vi "ziGetValueComplex.vi"(3 "error in":errorcluster, 4 "Path":string, 5 "Handle in":T1 {"Handle" format="0x%08x"; "Conn" format="0x%08x"}) -> (0 "error out":errorcluster, 1 "Value":cdb, 2 "Handle out":T1 {"Handle" format="0x%08x"; "Conn" format="0x%08x"})   [LabVIEW 2019, in "Zurich Instruments LabOne.lvlib"]
doc: "This vi retrieves the numerical value of the specified node as an double-type value. The vi returns the value first found that matches Path if more than one value is available (a wildcard is used in the Path)."
uses:
  Zurich Instruments LabOne.lvlib
  ziTypeHandle.ctl
  Private/ziLV64.dll
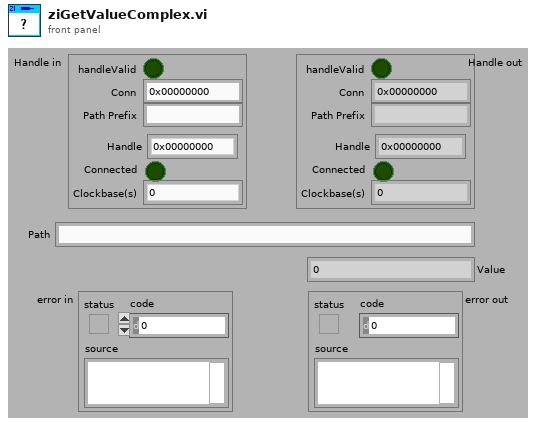
[diagram p1: front panel]
types:
  T1 = typedef "Zurich Instruments LabOne.lvlib/ziTypeHandle.ctl" = cluster{"handleValid":bool, "Conn":u64, "Path Prefix":string, "Handle":u64, "Connected":bool, "Clockbase(s)":dbl}
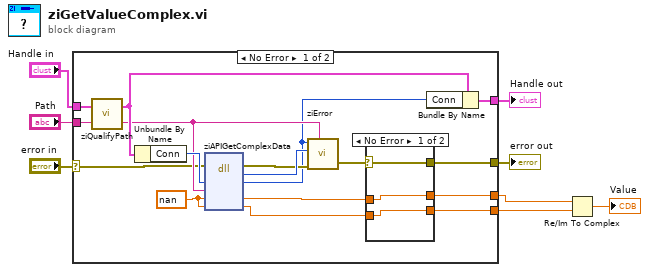
[diagram p0: block diagram]
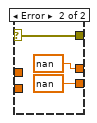
[diagram p2: hidden frame]
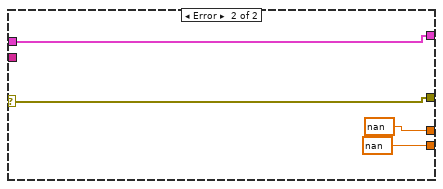
[diagram p3: hidden frame]
diagram:
  n1 = case shown="No Error" "error in" {
    selector: "error in" -> [w16 w35]
    tunnel: [w12 nan ("Value")] -> w2
    tunnel: [w14 w35] -> w8
    tunnel: [w22 w34] -> w7
    tunnel: "Handle in" -> [w21 w34]
    tunnel: "Path" -> [w20 _]
    tunnel: [w9 nan ("Value")] -> w3
    frame No Error {
      w11 = nan ("Value")
      n2 = call "ziQualifyPath.vi"("Path In"=w20, "Handle In"=w21) -> ("Path Out"=w18:string, "Handle Out"=w19:T1)
      n3 = Unbundle By Name(w19) -> ("Conn"=w25:u64)
      n4 = dll-call lib="D:/software/CryoTUM_14122020/CryoTUM/sub_vi-s/Equipment/Zurich Instruments LabOne/Private/ziLV*.*" fn="ziAPIGetComplexData"(error in=w16, "Conn"=w25, "Path"=w18, "ValueR"=w11, "ValueI"=w11) -> (error out=w23:errorcluster, "return type"=w24:u32, "Conn"=w17:u64, "ValueR"=w13:dbl, "ValueI"=w10:dbl)  [unwired: 2 in, 2 out]
      n5 = call "ziError.vi"("Conn"=w17, "ziErrorCode"=w24, "Error In"=w23, "Annotation"=w18) -> ("Error Out"=w15:errorcluster)  [unwired: 1 in, 1 out]
      n6 = case shown="No Error" w15 {
        selector: w15 -> [w28 w31]
        tunnel: [w28 w31] -> w14
        tunnel: w13 -> [w26 _]
        tunnel: [w27 nan ("Value")] -> w12
        tunnel: w10 -> [w27 _]
        tunnel: [w26 nan ("Value")] -> w9
        frame No Error {
        }
        frame Error {
        }
      }
      n7 = Bundle By Name(cluster=w19, "Conn"=w17) -> (w22:T1)
    }
    frame Error {
    }
  }
  "Handle out" <- w7
  "error out" <- w8
  n8 = Re/Im To Complex(1:w2, 2:w3) -> (0:→"Value":cdb)
